vi "Authenticate with Token.vi"(5 "Base URL":string, 6 "Body Parameters":T3[](array[typedef]), 7 "HTTP Method":T4, 8 "error in (no error)":errorcluster, 9 "Header Parameters":T3[](array[typedef]), 10 "URL Parameters":T3[](array[typedef]), 11 "OAuth Credentials":T1={"Consumer Key"="", "Signature Method"=enum."HMAC-SHA1", "Token"="", "Version"="", "Token Secret"="", "Consumer Secret"=""}) -> (0 "error out":errorcluster, 1 "Header Value":string, 2 "Header Parameter":string, 3 "Full URL":string, 4 "Body":string)   [LabVIEW 2011, in "i3-oauth.lvlib"]
doc: "Takes parameters used for authenticated requests and creates the Auth HTTP Header Parameter and Value, performs x-www-form-urlencoding of Body Parameters, and adds url parameters to the base url to form the full url. \n\nAll parameters added to this VI (Body Parameters, URL Parameters, and Header Parameters) will be included in the OAUTH signature in addition to the access token and consumer token, etc. Please read the API specification of the service being utilized to see which parameters should be included.\n\nExample:\nThe Twitter API v1.1 requires that when performing a POST that the status be added as a parameter to the body and included as part of the OAUTH signature. In this case the status is wired to the Body parameter of this function, it is used as part of the signature, and the x-www-form-urlencoded version of the body parameters are returned to send to Twitter. Alternatively the Twitter media multipart post specifies that the status and image are NOT added to the body so in this case the user will not include them as part of the signature and has to manually create the Post body"
uses:
  i3-oauth.lvlib
  Controls/key-value-pairs.ctl
  Controls/HTTP Method.ctl
  Controls/OAuth Credentials.ctl
  Controls/Signature Method.ctl
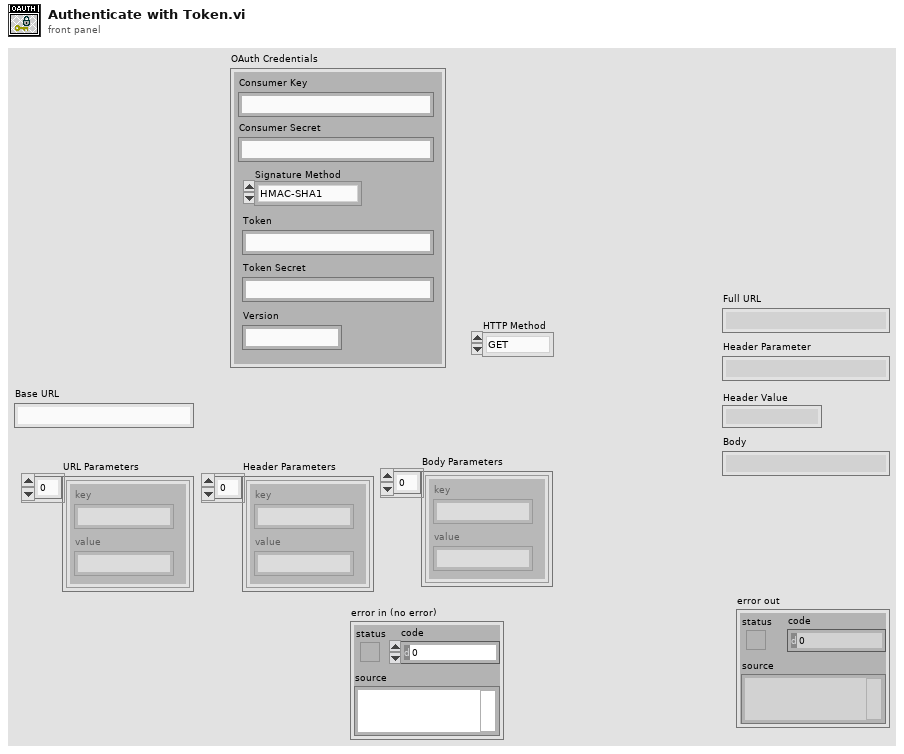
[diagram p1: front panel]
types:
  T1 = typedef "i3-oauth.lvlib/OAuth Credentials.ctl" = cluster{"Consumer Key":string, "Signature Method":T2, "Token":string, "Version":string, "Token Secret":string, "Consumer Secret":string}
  T2 = typedef "i3-oauth.lvlib/Signature Method.ctl" = enum16{"HMAC-MD5", "HMAC-SHA1", "HMAC-SHA224", "HMAC-SHA256", "HMAC-SHA384", "HMAC-SHA512"}
  T3 = typedef "i3-oauth.lvlib/key-value-pairs.ctl" = cluster{"key":string, "value":string}
  T4 = typedef "i3-oauth.lvlib/HTTP Method.ctl" = enum16{"GET", "POST", "PUT", "DELETE"}
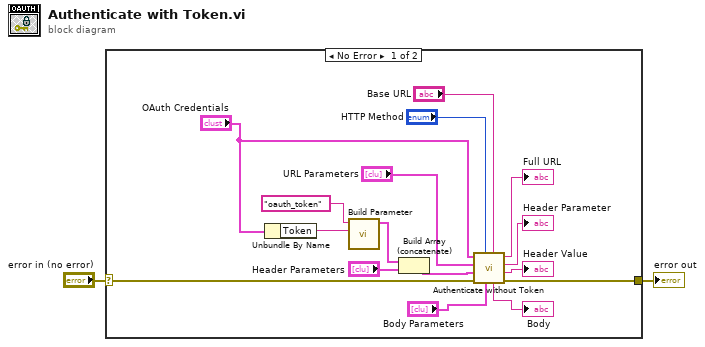
[diagram p0: block diagram]
diagram:
  n1 = case shown="No Error" "error in (no error)" {
    selector: "error in (no error)" -> [w14 w19]
    tunnel: [w15 w19] -> w2
    frame No Error {
      n2 = Unbundle By Name("OAuth Credentials") -> ("Token"=w10:string)
      n3 = call "Build Parameter.vi"("Value"=w10, "Key"="oauth_token") -> ("Parameter Array"=w6:T3[])  [unwired: 9 in]
      n4 = Build Array (concatenate)(w6, "Header Parameters") -> (w8:T3[])
      n5 = call "Authenticate without Token.vi"("Base URL"="Base URL", "Body Parameters"="Body Parameters", "HTTP Method"="HTTP Method", "error in (no error)"=w14, "Header Parameters"=w8, "URL Parameters"="URL Parameters", "OAuth Credentials"="OAuth Credentials") -> ("error out"=w15:errorcluster, "Header Value"=→"Header Value":string, "Header Parameter"=→"Header Parameter":string, "Full URL"=→"Full URL":string, "Body"=→"Body":string)
    }
    frame Error {
    }
  }
  "error out" <- w2
